vi "AlliGator Get (Smoothed) Gate Images Sum & Stack.vi"(6 "Phasor Plot Smoothing Options":T1={"Use Phasor Plot Smoothing"=FALSE, "Kernel Type"=enum."Uniform", "Bin"=1, "Algorithm"=enum."Rapid"} {"Bin" min=1 step=2}, 7 "Optional Rectangle":i32[](array[numeric]), 8 "Error In":errorcluster, 9 "Pixel Counts Constraints":T4 {"High Count Pixels Rejection Options"."High Percentile" min=0.0 max=100.0; "Low Count Pixels Rejection Options"."Low Percentile" min=0.0 max=100.0}, 10 "Sum Image":T7, 11 "Image Array":T7[](array[typedef])) -> (0 "Error Out":errorcluster, 1 "[[Valid Pixel]] VxH Array":bool[][](array[boolean]), 2 "Gate Images Stack (N xV xH)":sgl[][][](array[numeric]), 3 "Sum Image (VxH)":sgl[][](array[numeric]), 4 "Message":string)   [LabVIEW 2021, in "AlliGator Phasor Plot.lvlib"]
doc: "Computes the smoothed array of gate image data for subsequent phasor plot calculation."
uses:
  AlliGator Phasor Plot.lvlib
  Time/Time.lvlib
  Arrays/Arrays.lvlib
  <vilib>/ErrorRing/Error Ring.xnode
  <vilib>/Utility/error.llb/Error Cluster From Error Code.vi
  AlliGator Abort.vi
  AlliGator Globals, Variables & Constants.lvlib
  <vilib>/vision/EDVR.llb/IMAQ ImageToEDVR 2D U8.vi
  <vilib>/vision/EDVR.llb/IMAQ ImageToEDVR 2D I16.vi
  <vilib>/vision/EDVR.llb/IMAQ ImageToEDVR 2D SGL.vi
  <vilib>/vision/EDVR.llb/IMAQ ImageToEDVR 2D U16.vi
  Utilities/Utilities.lvlib
  <vilib>/vision/Image Controls.llb/IMAQ Image.ctl
  Arrays/Kernel Type.ctl
  AlliGator Low Count Pixels Rejection Options.ctl
  AlliGator Settings.lvlib
  AlliGator High Count Pixels Rejection Options.ctl
  AlliGator Pixel Counts Constraints.ctl
  Arrays/Smoothing Algorithm.ctl
  AlliGator Phasor Plot Smoothing Options.ctl
panel:
  out "CPU (s)":dbl
  # "see the AlliGator License on the block diagram (Ctrl+E or Window:Show Block Diagram)"
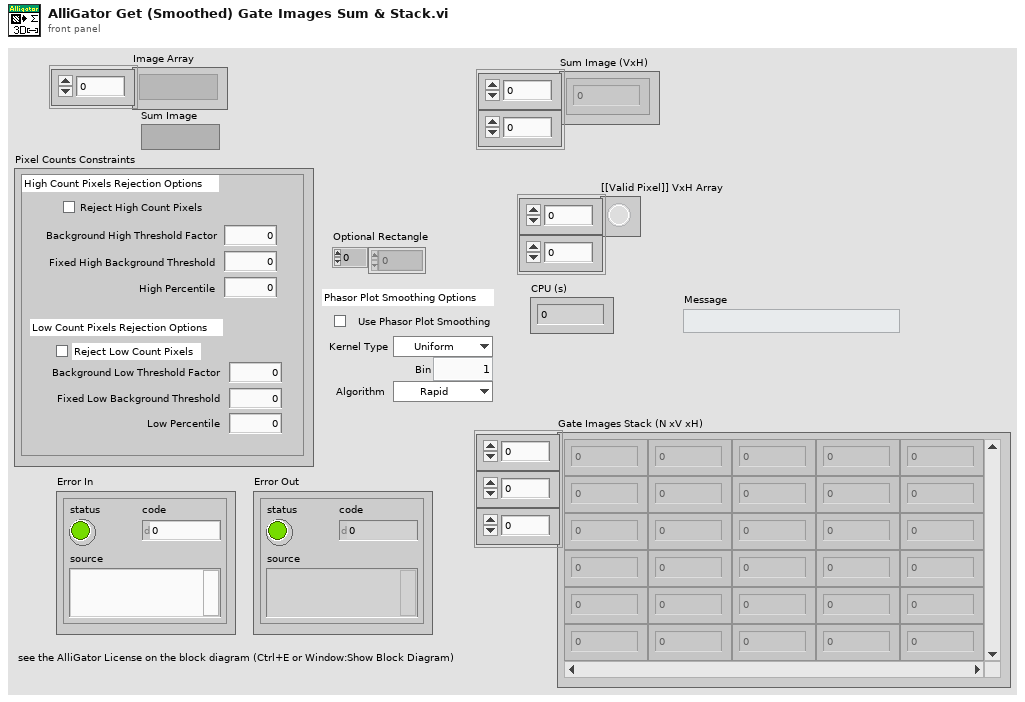
[diagram p1: front panel]
types:
  T1 = typedef "AlliGator Phasor Plot.lvlib/AlliGator Phasor Plot Smoothing Options.ctl" = cluster{"Use Phasor Plot Smoothing":bool, "Kernel Type":T2, "Bin":i32, "Algorithm":T3}
  T2 = typedef "Arrays.lvlib/Kernel Type.ctl" = enum16{"Uniform", "Bilinear", "Gaussian"}
  T3 = typedef "Arrays.lvlib/Smoothing Algorithm.ctl" = enum16{"Rapid", "Thorough"}
  T4 = typedef "AlliGator Settings.lvlib/AlliGator Pixel Counts Constraints.ctl" = cluster{"High Count Pixels Rejection Options":T5, "Low Count Pixels Rejection Options":T6}
  T5 = typedef "AlliGator Settings.lvlib/AlliGator High Count Pixels Rejection Options.ctl" = cluster{"Background High Threshold Factor":dbl, "Fixed High Background Threshold":dbl, "Reject High Count Pixels":bool, "High Percentile":dbl}
  T6 = typedef "AlliGator Settings.lvlib/AlliGator Low Count Pixels Rejection Options.ctl" = cluster{"Background Low Threshold Factor":dbl, "Fixed Low Background Threshold":dbl, "Reject Low Count Pixels":bool, "Low Percentile":dbl}
  T7 = typedef "IMAQ Image.ctl" = refnum<image>
  T8 = typedef "Image Type" = u32
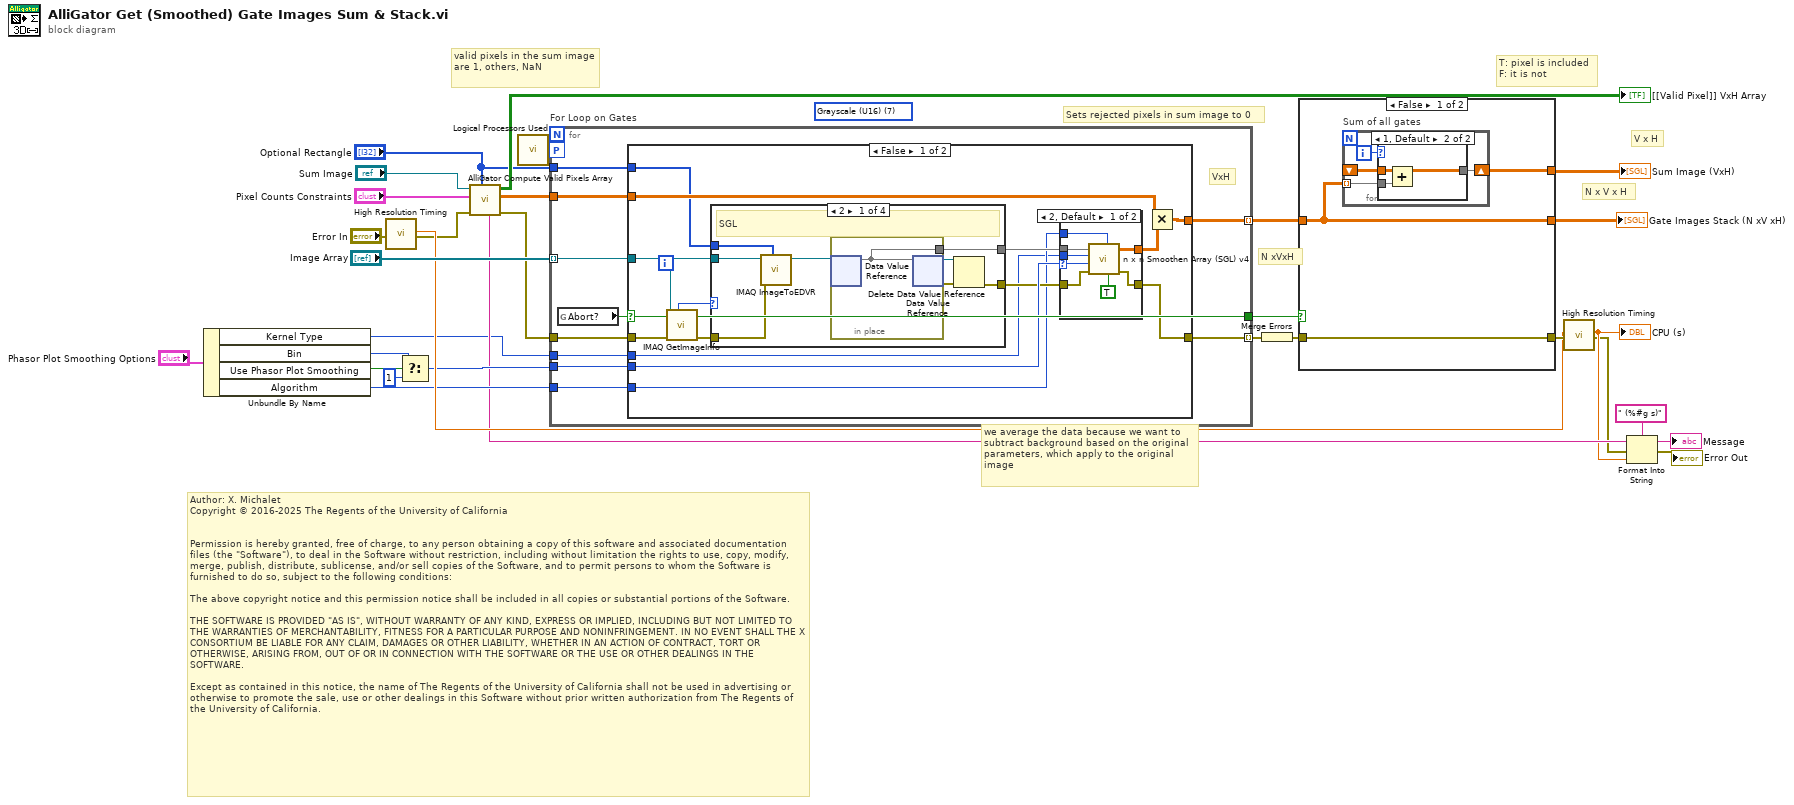
[diagram p0: block diagram]
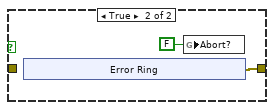
[diagram p3: hidden frame]
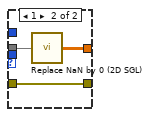
[diagram p4: hidden frame]
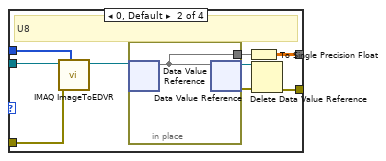
[diagram p5: hidden frame]
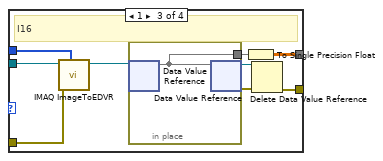
[diagram p6: hidden frame]
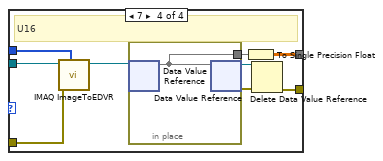
[diagram p7: hidden frame]
diagram:
  (unwired) T8 7 items=["Grayscale (U8)", "Grayscale (I16)", "Grayscale (SGL)", "Complex (CSG)", "RGB (U32)", "HSL (U32)", "RGB (U64)", "Grayscale (U16)"] ("Image Type")
  # "Author: X. Michalet\nCopyright © 2016-2025 The Regents of the University of California\n \n\nPermission is hereby granted, free of charge, to any person obtaining a copy of this software and associated documentation files (the \"Software\"), to deal in the Software without restriction, including without limitation the rights to use, copy, modify, merge, publish, distribute, sublicense, and/or sell copies of the Software, and to permit persons to whom the Software is furnished to do so, subject to the following conditions:\n\nThe above copyright notice and this permission notice shall be included in all copies or substantial portions of the Software.\n\nTHE SOFTWARE IS PROVIDED \"AS IS\", WITHOUT WARRANTY OF ANY KIND, EXPRESS OR IMPLIED, INCLUDING BUT NOT LIMITED TO THE WARRANTIES OF MERCHANTABILITY, FITNESS FOR A PARTICULAR PURPOSE AND NONINFRINGEMENT. IN NO EVENT SHALL THE X CONSORTIUM BE LIABLE FOR ANY CLAIM, DAMAGES OR OTHER LIABILITY, WHETHER IN AN ACTION OF CONTRACT, TORT OR OTHERWISE, ARISING FROM, OUT OF OR IN CONNECTION WITH THE SOFTWARE OR THE USE OR OTHER DEALINGS IN THE SOFTWARE.\n\nExcept as contained in this notice, the name of The Regents of the University of California shall not be used in advertising or otherwise to promote the sale, use or other dealings in this Software without prior written authorization from The Regents of the University of California."
  # "N xVxH"
  # "valid pixels in the sum image are 1, others, NaN"
  # "Sets rejected pixels in sum image to 0"
  # "T: pixel is included\nF: it is not"
  # "we average the data because we want to subtract background based on the original parameters, which apply to the original image"
  # "N x V x H"
  # "V x H"
  n1 = Unbundle By Name("Phasor Plot Smoothing Options") -> ("Kernel Type"=w5:T2, "Bin"=w16:i32, "Use Phasor Plot Smoothing"=w17:bool, "Algorithm"=w13:T3)
  n2 = call "High Resolution Timing.vi"("Error In"="Error In") -> ("elapsed (relative) seconds"=w28:dbl, "Error Out"=w26:errorcluster)  [unwired: 16 in, 1 out]
  n3 = Select(t=w16, s=w17, f=1) -> (s? t:f=w14:i32)
  n4 = call "AlliGator Compute Valid Pixels Array.vi"("Optional Rectangle"="Optional Rectangle", "error in (no error)"=w26, "Pixel Counts Constraints"="Pixel Counts Constraints", "Sum Image"="Sum Image") -> ("error out"=w22:errorcluster, "[[Valid Pixel (1,NaN)]] VxH Array"=w20:sgl[][], "[[Valid Pixel]] VxH Array"=→"[[Valid Pixel]] VxH Array":bool[][], "Message"=w11:string)  [unwired: 3 in, 1 out]
  n5 = call "Logical Processors Used.vi"() -> ("# Logical Processor Used"=w1:i32)  [unwired: 6 in]
  n6 = for "For Loop on Gates" {
    tunnel: "Image Array" -> [w38] mode=indexing
    tunnel: w20 -> [w39]
    tunnel: [w40] -> w4 mode=indexing
    tunnel: w14 -> [w37]
    tunnel: w22 -> [w41]
    tunnel: [w36] -> w23 mode=indexing
    tunnel: [w35] -> w19
    tunnel: w13 -> [w34]
    tunnel: "Optional Rectangle" -> [w33]
    tunnel: w5 -> [w32]
    workers-P: w1 -> [_]
    # "VxH"
    n7 = global read "AlliGator Abort.vi" "Abort?"() -> (w35:bool)
    n8 = case shown="False" w35 {
      tunnel: w41 -> [w55 w106]
      tunnel: [w53 w107] -> w40
      tunnel: w39 -> [w45 w107]
      tunnel: w38 -> [w51 _]
      tunnel: w37 -> [w50 _]
      tunnel: [w47 w106] -> w36
      tunnel: w34 -> [w44 _]
      tunnel: w33 -> [w43 _]
      tunnel: w32 -> [w42 _]
      frame False {
        n9 = call "IMAQ GetImageInfo"("error in (no error)"=w55, "Image"=w51) -> ("error out"=w52:errorcluster, "Image Type"=w54:T8)  [unwired: 2 in, 6 out]
        n10 = case shown="2" w54 {
          tunnel: [w71 w77 w87 w97] -> w46
          tunnel: w51 -> [w74 w84 w94 w104]
          tunnel: w52 -> [w73 w83 w93 w103]
          tunnel: [w68 w78 w88 w98] -> w48
          tunnel: w43 -> [w67 w76 w86 w96]
          frame 2 {
            # "SGL"
            n11 = call-poly <vilib>:"IMAQ ImageToEDVR.vi"("Optional Rectangle"=w67, "error in (no error)"=w73, "Image"=w74) -> ("EDVR 2D SGL"=w72:refnum<data-value>)  [unwired: 6 in, 2 out]
            n12 = in-place {
              in-place-border: [w75] -> w71
              n13 = in-place-dvr #1(w72) -> (w75:sgl[][])  [unwired: 1 out]
              n14 = in-place-dvr #1(w75) -> (w70:refnum<data-value>, w69:errorcluster)
            }
            n15 = Delete Data Value Reference(data value reference=w70, error in=w69) -> (error out=w68:errorcluster)  [unwired: 1 out]
          }
          frame 0, Default {
            # "U8"
            n16 = call-poly <vilib>:"IMAQ ImageToEDVR.vi"("Optional Rectangle"=w76, "error in (no error)"=w83, "Image"=w84) -> ("EDVR 2D U8"=w82:refnum<data-value>)  [unwired: 6 in, 2 out]
            n17 = in-place {
              in-place-border: [w85] -> w81
              n18 = in-place-dvr #2(w82) -> (w85:u8[][])  [unwired: 1 out]
              n19 = in-place-dvr #2(w85) -> (w80:refnum<data-value>, w79:errorcluster)
            }
            n20 = To Single Precision Float(number=w81) -> (single precision float=w77:sgl[][])
            n21 = Delete Data Value Reference(data value reference=w80, error in=w79) -> (error out=w78:errorcluster)  [unwired: 1 out]
          }
          frame 1 {
            # "I16"
            n22 = call-poly <vilib>:"IMAQ ImageToEDVR.vi"("Optional Rectangle"=w86, "error in (no error)"=w93, "Image"=w94) -> ("EDVR 2D I16"=w92:refnum<data-value>)  [unwired: 6 in, 2 out]
            n23 = in-place {
              in-place-border: [w95] -> w91
              n24 = in-place-dvr #3(w92) -> (w95:i16[][])  [unwired: 1 out]
              n25 = in-place-dvr #3(w95) -> (w90:refnum<data-value>, w89:errorcluster)
            }
            n26 = To Single Precision Float(number=w91) -> (single precision float=w87:sgl[][])
            n27 = Delete Data Value Reference(data value reference=w90, error in=w89) -> (error out=w88:errorcluster)  [unwired: 1 out]
          }
          frame 7 {
            # "U16"
            n28 = call-poly <vilib>:"IMAQ ImageToEDVR.vi"("Optional Rectangle"=w96, "error out"=w103, "Image"=w104) -> ("EDVR 2D U16"=w102:refnum<data-value>)  [unwired: 6 in, 2 out]
            n29 = in-place {
              in-place-border: [w105] -> w101
              n30 = in-place-dvr #4(w102) -> (w105:u16[][])  [unwired: 1 out]
              n31 = in-place-dvr #4(w105) -> (w100:refnum<data-value>, w99:errorcluster)
            }
            n32 = To Single Precision Float(number=w101) -> (single precision float=w97:sgl[][])
            n33 = Delete Data Value Reference(data value reference=w100, error in=w99) -> (error out=w98:errorcluster)  [unwired: 1 out]
          }
        }
        n34 = case shown="2, Default" w50 {
          selector: w50 -> [w61 _]
          tunnel: w46 -> [w63 w66]
          tunnel: [w62 w64] -> w49
          tunnel: w48 -> [w60 w65]
          tunnel: [w59 w65] -> w47
          tunnel: w42 -> [w58 _]
          tunnel: w44 -> [w56 _]
          frame 2, Default {
            n35 = call "n x n Smoothen Array (SGL) v4.vi"("Average"=TRUE, "Algorithm"=w56, "Error In"=w60, "Kernel Size"=w61, "Kernel Type"=w58, "Array in"=w63) -> ("Error Out"=w59:errorcluster, "Array out"=w62:sgl[][])  [unwired: 3 in, 1 out]
          }
          frame 1 {
            n36 = call "Replace NaN by 0 (2D SGL).vi"("Array in"=w66) -> ("Array out"=w64:sgl[][])  [unwired: 8 in]
          }
        }
        n37 = Multiply(x=w45, y=w49) -> (x*y=w53:sgl[][])
      }
      frame True {
      }
    }
  }
  n38 = Merge Errors(w23) -> (w21:errorcluster)
  n39 = case shown="False" w19 {
    tunnel: w21 -> [w110 _]
    tunnel: [w110 w120] -> w30
    tunnel: w4 -> [w108 _]
    tunnel: [w109 _] -> w3
    tunnel: [w108 _] -> w2
    frame False {
      n40 = for "Sum of all gates" {
        tunnel: w108 -> [w113] mode=indexing
        shift-right: [w112] -> w109
        shift-left: _ -> [w111]
        i -> [w114]
        n41 = case shown="1, Default" w114 {
          tunnel: w113 -> [w115 w117]
          tunnel: [w115 w116] -> w112
          tunnel: w111 -> [_ w118]
          frame 0 {
          }
          frame 1, Default {
            n42 = Add(x=w118, y=w117) -> (x+y=w116:sgl[][])
          }
        }
      }
    }
    frame True {
      n43 = xnode "Error Ring"() -> ("error out"=w120:errorcluster)
      n44 = global write "AlliGator Abort.vi" "Abort?"(FALSE ("Abort?")) -> ()
    }
  }
  "Sum Image (VxH)" <- w3
  "Gate Images Stack (N xV xH)" <- w2
  n45 = call "High Resolution Timing.vi"("relative seconds (NaN)"=w28, "Error In"=w30) -> ("elapsed (relative) seconds"=w8:dbl, "Error Out"=w7:errorcluster)  [unwired: 15 in, 1 out]
  "CPU (s)" <- w8
  n46 = Format Into String(format string=" (%#g s)", initial string=w11, error in=w7, w8) -> (resulting string=→"Message":string, error out=→"Error Out":errorcluster)
